vi "call module.vi"() -> ()   [LabVIEW 2023]
uses:
  <extravilib>/ChannelInstances/Messenger-t'Message Queue.lvlib-Message Cluster.ctl'/Instantiate.vi
  <vilib>/DLR/CMH Lib/Message Queue/Enqueue Multiple Messages.vi
  Camera Calibration.lvlib
  <vilib>/DLR/CMH Lib/Message Queue.lvlib
panel:
  out "message":string
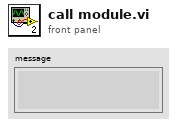
[diagram p1: front panel]
types:
  T1 = typedef "IMAQ Image.ctl" = refnum<image>
  T2 = typedef "Messenger-t'Message Queue.lvlib-Message Cluster.ctl'.lvlib/))Channel.ctl" = refnum<queue>
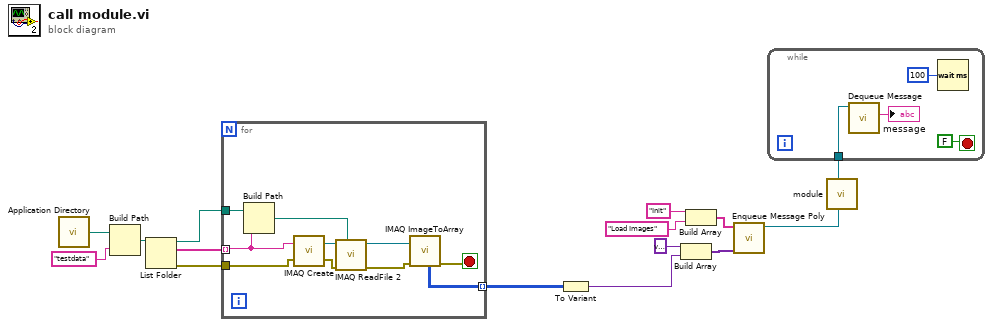
[diagram p0: block diagram]
diagram:
  n1 = call <vilib>:"Application Directory.vi"() -> ("Application Directory"=w10:path)
  n2 = Build Path(base path=w10, name or relative path="testdata") -> (appended path=w8:path)
  n3 = List Folder(path=w8) -> (path out=w7:path, filenames=w9:string[], error out=w2:errorcluster)  [unwired: 3 in, 1 out]
  n4 = for {
    tunnel: w9 -> [w21] mode=indexing
    tunnel: w7 -> [w25]
    tunnel: [w18] -> w4 mode=indexing
    tunnel: w2 -> [w16]
    stop <- w17 stop-if-true
    n5 = Build Path(base path=w25, name or relative path=w21) -> (appended path=w24:path)
    n6 = call "IMAQ Create"("Image Name"=w21, "error in (no error)"=w16) -> ("New Image"=w23:T1, "error out"=w22:errorcluster)  [unwired: 3 in]
    n7 = call "IMAQ ReadFile 2"("File Path"=w24, "error in (no error)"=w22, "Image"=w23) -> ("error out"=w19:errorcluster, "Image Out"=w20:T1)  [unwired: 4 in, 3 out]
    n8 = call "IMAQ ImageToArray"("error in (no error)"=w19, "Image"=w20) -> ("Image Pixels (U16)"=w18:u16[][], "error out"=w17:errorcluster)  [unwired: 2 in, 3 out]
  }
  n9 = To Variant(anything=w4) -> (Variant=w3:variant)
  n10 = Build Array(variant, w3) -> (w6:variant[])
  n11 = Build Array("Init" ("Message"), "Load Images" ("element")) -> (w12:string[])
  n12 = call-poly <vilib>:"Enqueue Message Poly.vi"("data array"=w6, "cmd array"=w12) -> ("channel"=w14:T2)  [unwired: 9 in]
  n13 = call "module.vi"("cmd channel"=w14) -> ("response"=w13:T2)  [unwired: 10 in]
  n14 = while {
    tunnel: w13 -> [w27]
    stop <- FALSE stop-if-true
    n15 = call <vilib>:"Dequeue Message.vi"("channel"=w27) -> ("message"=→"message":string)  [unwired: 8 in, 2 out]
    n16 = Wait (ms)(milliseconds to wait=u32 100) -> ()  [unwired: 1 out]
  }
